vi "Launch Subordinate and Add.vi"(6 "Position":T1, 8 "error in":errorcluster, 9 "Panel Definiton":T2, 10 "Identifier":string, 11 "Base Software in":refnum<class "Base Software.lvclass">) -> (0 "error out":errorcluster, 3 "Base Software out":refnum<class "Base Software.lvclass">)   [LabVIEW 2019, in "Base Software.lvlib" / "Main.lvlib" / "Base Software.lvclass"]
uses:
  Project/Base Software.lvclass
  builds/Engine/Panel Manager.lvlibp/Panel Actor/Panel Actor.lvclass
  builds/Engine/Panel.lvlibp/Panel/Panel.lvclass
  Custom Controls/Panel_Positions.ctl
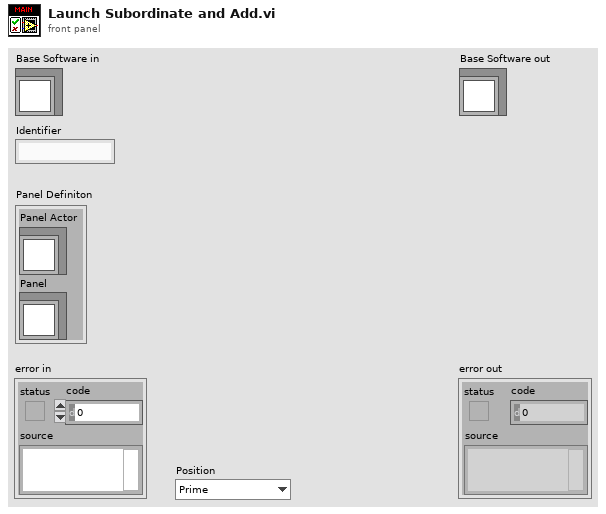
[diagram p1: front panel]
types:
  T1 = typedef "Base Software.lvlib/Main.lvlib/Base Software.lvclass/Panel_Positions.ctl" = enum16{"Prime", "Right", "Bottom", "Left", "Mission"}
  T2 = cluster{"Panel Actor":refnum<class "Panel Actor.lvclass">, "Panel":refnum<class "Panel.lvclass">}
  T3 = typedef "Base Software.lvlib/Main.lvlib/Base Software.lvclass/Subordinate.ctl" = cluster{"Identifier":string, "Enqueuer":refnum<class "Message Enqueuer.lvclass">, "Position":T1}
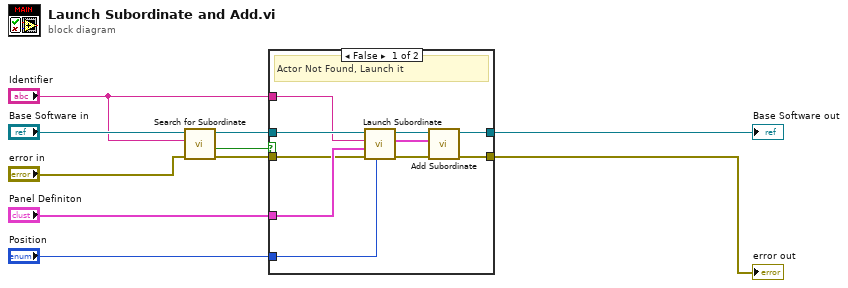
[diagram p0: block diagram]
diagram:
  n1 = call "Search for Subordinate.vi"("error in"="error in", "Identifier"="Identifier", "Base Software in"="Base Software in") -> ("error out"=w9:errorcluster, "Found"=w2:bool, "Base Software out"=w8:refnum<class "Base Software.lvclass">)  [unwired: 3 in, 3 out]
  n2 = case shown="False" w2 {
    tunnel: "Panel Definiton" -> [w20 _]
    tunnel: w9 -> [w19 w21]
    tunnel: w8 -> [w15 w22]
    tunnel: [w14 w22] -> w7
    tunnel: "Identifier" -> [w13 _]
    tunnel: [w12 w21] -> w3
    tunnel: "Position" -> [w11 _]
    frame False {
      # "Actor Not Found, Launch it"
      n3 = call "Launch Subordinate.vi"("Position"=w11, "error in"=w19, "Panel Definiton"=w20, "Identifier"=w13, "Base Software in"=w15) -> ("error out"=w18:errorcluster, "Subordinate"=w17:T3, "Base Software out"=w16:refnum<class "Base Software.lvclass">)  [unwired: 4 in]
      n4 = call "Add Subordinate.vi"("error in"=w18, "Subordinate"=w17, "Base Software in"=w16) -> ("error out"=w12:errorcluster, "Base Software out"=w14:refnum<class "Base Software.lvclass">)  [unwired: 7 in]
    }
    frame True {
      # "Actor Already Launched"
    }
  }
  "error out" <- w3
  "Base Software out" <- w7
